vi "clean-kinetics-SD.vi"(5 "timedelays":dbl[](array[numeric]), 6 "kinetics":dbl[](array[numeric]), 7 "Data":dbl[][](array[numeric]), 8 "bounds":cluster{"minY":dbl, "maxY":dbl}, 9 "Clean mode":enum32{"delete", "approx"}(radio)=enum."approx", 10 "TDpixels":cluster{"minY":i32, "maxY":i32}) -> (1 "Data out":dbl[][](array[numeric]), 2 "timedelays out":dbl[](array[numeric]))   [LabVIEW 2020]
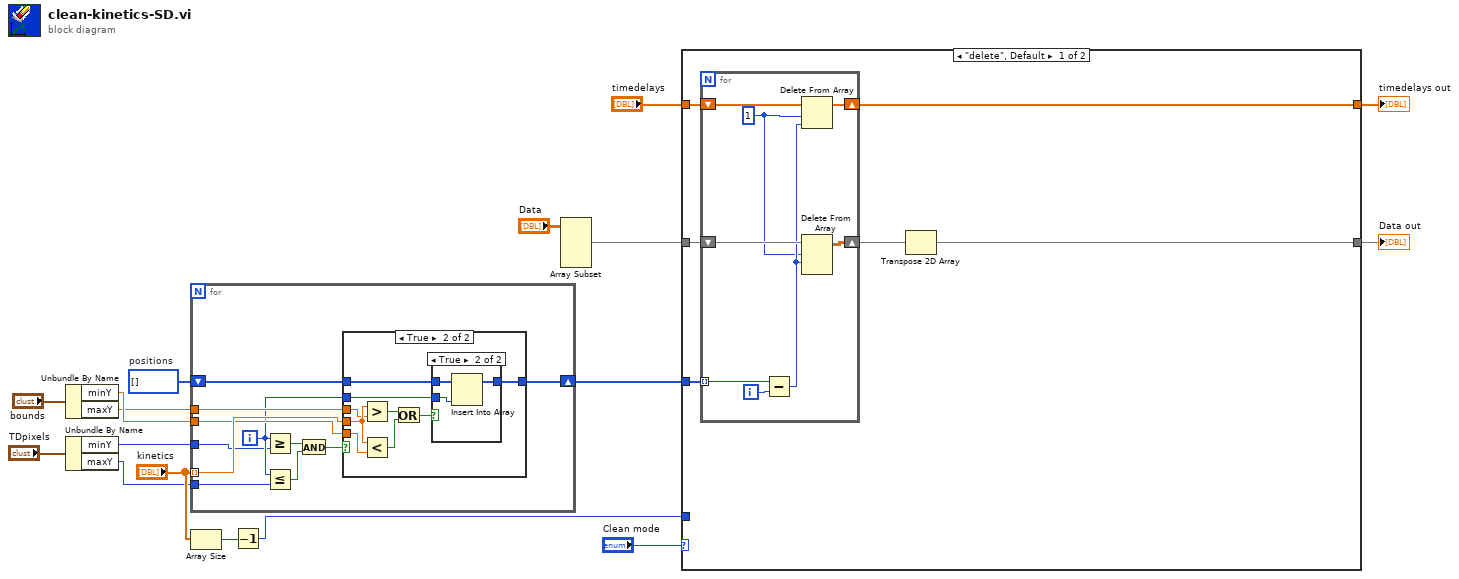
[diagram p0: block diagram]
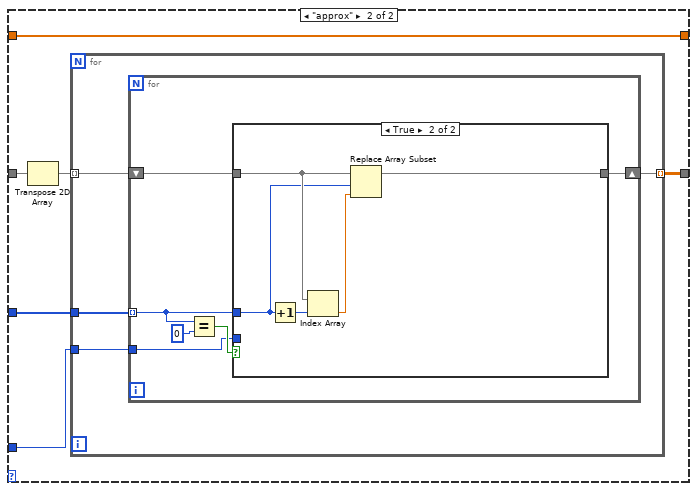
[diagram p2: hidden frame]
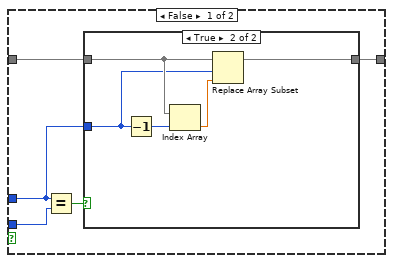
[diagram p3: hidden frame]
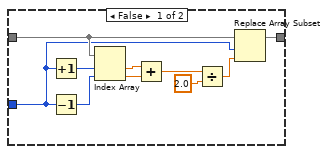
[diagram p4: hidden frame]
diagram:
  w17 = i32[] []  # positions
  n1 = Unbundle By Name("bounds") -> ("minY"=w6:dbl, "maxY"=w5:dbl)
  n2 = Unbundle By Name("TDpixels") -> ("minY"=w2:i32, "maxY"=w3:i32)
  n3 = for {
    tunnel: "kinetics" -> [w28] mode=indexing
    shift-right: [w26] -> w15
    shift-left: w17 -> [w27]
    tunnel: w6 -> [w25]
    tunnel: w5 -> [w24]
    tunnel: w3 -> [w23]
    tunnel: w2 -> [w21]
    i -> [w22]
    n4 = Greater Or Equal?(x=w22, y=w21) -> (x >= y?=w20:bool)
    n5 = Less Or Equal?(x=w22, y=w23) -> (x <= y?=w19:bool)
    n6 = And(x=w20, y=w19) -> (x .and. y?=w18:bool)
    n7 = case shown="True" w18 {
      tunnel: w28 -> [_ w38]
      tunnel: w22 -> [_ w35]
      tunnel: w27 -> [w29 w34]
      tunnel: [w29 w33] -> w26
      tunnel: w25 -> [_ w31]
      tunnel: w24 -> [_ w30]
      frame False {
      }
      frame True {
        n8 = Greater?(x=w38, y=w30) -> (0:w37:bool)
        n9 = Less?(x=w38, y=w31) -> (x < y?=w36:bool)
        n10 = Or(x=w37, y=w36) -> (x .or. y?=w32:bool)
        n11 = case shown="True" w32 {
          tunnel: w35 -> [_ w41]
          tunnel: w34 -> [w39 w42]
          tunnel: [w39 w40] -> w33
          frame False {
          }
          frame True {
            n12 = Insert Into Array(array=w42, new element=w41) -> (w40:i32[])  [unwired: 1 in]
          }
        }
      }
    }
  }
  n13 = Array Size(array="kinetics") -> (size(s)=w10:i32)
  n14 = Decrement(x=w10) -> (x-1=w8:i32)
  n15 = Array Subset(array="Data") -> (w16:dbl[][])  [unwired: 4 in]
  n16 = case shown="\"delete\", Default" "Clean mode" {
    tunnel: w16 -> [w48 w61]
    tunnel: w15 -> [w47 w59]
    tunnel: "timedelays" -> [w46 w62]
    tunnel: [w45 w62] -> w12
    tunnel: [w43 w57] -> w9
    tunnel: w8 -> [_ w58]
    frame "delete", Default {
      n17 = for {
        shift-right: [w54] -> w44
        shift-left: w48 -> [w56]
        tunnel: w47 -> [w55] mode=indexing
        shift-right: [w51] -> w45
        shift-left: w46 -> [w52]
        i -> [w53]
        w49 = 1 ("length")
        n18 = Subtract(x=w55, y=w53) -> (x-y=w50:i32)
        n19 = Delete From Array(array=w52, length=w49, index=w50) -> (array with subset deleted=w51:dbl[])  [unwired: 1 out]
        n20 = Delete From Array(array=w56, length=w49, index (row)=w50) -> (array with subset deleted=w54:dbl[][])  [unwired: 1 in, 1 out]
      }
      n21 = Transpose 2D Array(2D array=w44) -> (transposed array=w43:dbl[][])
    }
    frame "approx" {
      n22 = Transpose 2D Array(2D array=w61) -> (transposed array=w60:dbl[][])
      n23 = for {
        tunnel: w60 -> [w64] mode=indexing
        tunnel: w59 -> [w66]
        tunnel: w58 -> [w65]
        tunnel: [w63] -> w57 mode=indexing
        n24 = for {
          tunnel: w66 -> [w70] mode=indexing
          tunnel: w65 -> [w69]
          shift-right: [w67] -> w63
          shift-left: w64 -> [w68]
          n25 = Equal?(x=w70, y=0) -> (x = y?=w71:bool)
          n26 = case shown="True" w71 {
            tunnel: w70 -> [w74 w94]
            tunnel: w69 -> [w77 _]
            tunnel: w68 -> [w75 w96]
            tunnel: [w73 w97] -> w67
            frame False {
              n27 = Equal?(x=w74, y=w77) -> (x = y?=w76:bool)
              n28 = case shown="True" w76 {
                tunnel: w75 -> [w87 w91]
                tunnel: w74 -> [w85 w90]
                tunnel: [w78 w92] -> w73
                frame False {
                  n29 = Increment(x=w85) -> (x+1=w86:i32)
                  n30 = Decrement(x=w85) -> (x-1=w84:i32)
                  n31 = Index Array(array=w87, index #1=w86, index #2=w84) -> (element #1=w83:dbl, element #2=w82:dbl)
                  n32 = Add(x=w83, y=w82) -> (x+y=w81:dbl)
                  n33 = Divide(x=w81, y=2.0) -> (x/y=w79:dbl)
                  n34 = Replace Array Subset(array=w87, new element=w79, index=w85) -> (w78:dbl[])
                }
                frame True {
                  n35 = Decrement(x=w90) -> (x-1=w89:i32)
                  n36 = Index Array(array=w91, index=w89) -> (element=w88:dbl)
                  n37 = Replace Array Subset(array=w91, new element=w88, index=w90) -> (w92:dbl[])
                }
              }
            }
            frame True {
              n38 = Increment(x=w94) -> (x+1=w93:i32)
              n39 = Index Array(array=w96, index=w93) -> (element=w95:dbl)
              n40 = Replace Array Subset(array=w96, new element=w95, index=w94) -> (w97:dbl[])
            }
          }
        }
      }
    }
  }
  "Data out" <- w9
  "timedelays out" <- w12
